vi "strain_fgv_config.vi"(8 "error in":errorcluster caption="에러 입력") -> (0 "error out":errorcluster caption="에러 출력", 3 "task out":refnum<k21> caption="태스크 출력")   [LabVIEW 2013]
uses:
  <vilib>/DAQmx/configure/timing.llb/DAQmx Timing (Sample Clock).vi
  <vilib>/DAQmx/create/channels.llb/DAQmx Create Channel (AI-Strain-Strain Gage).vi
  <resource>/objmgr/daqmx.rc
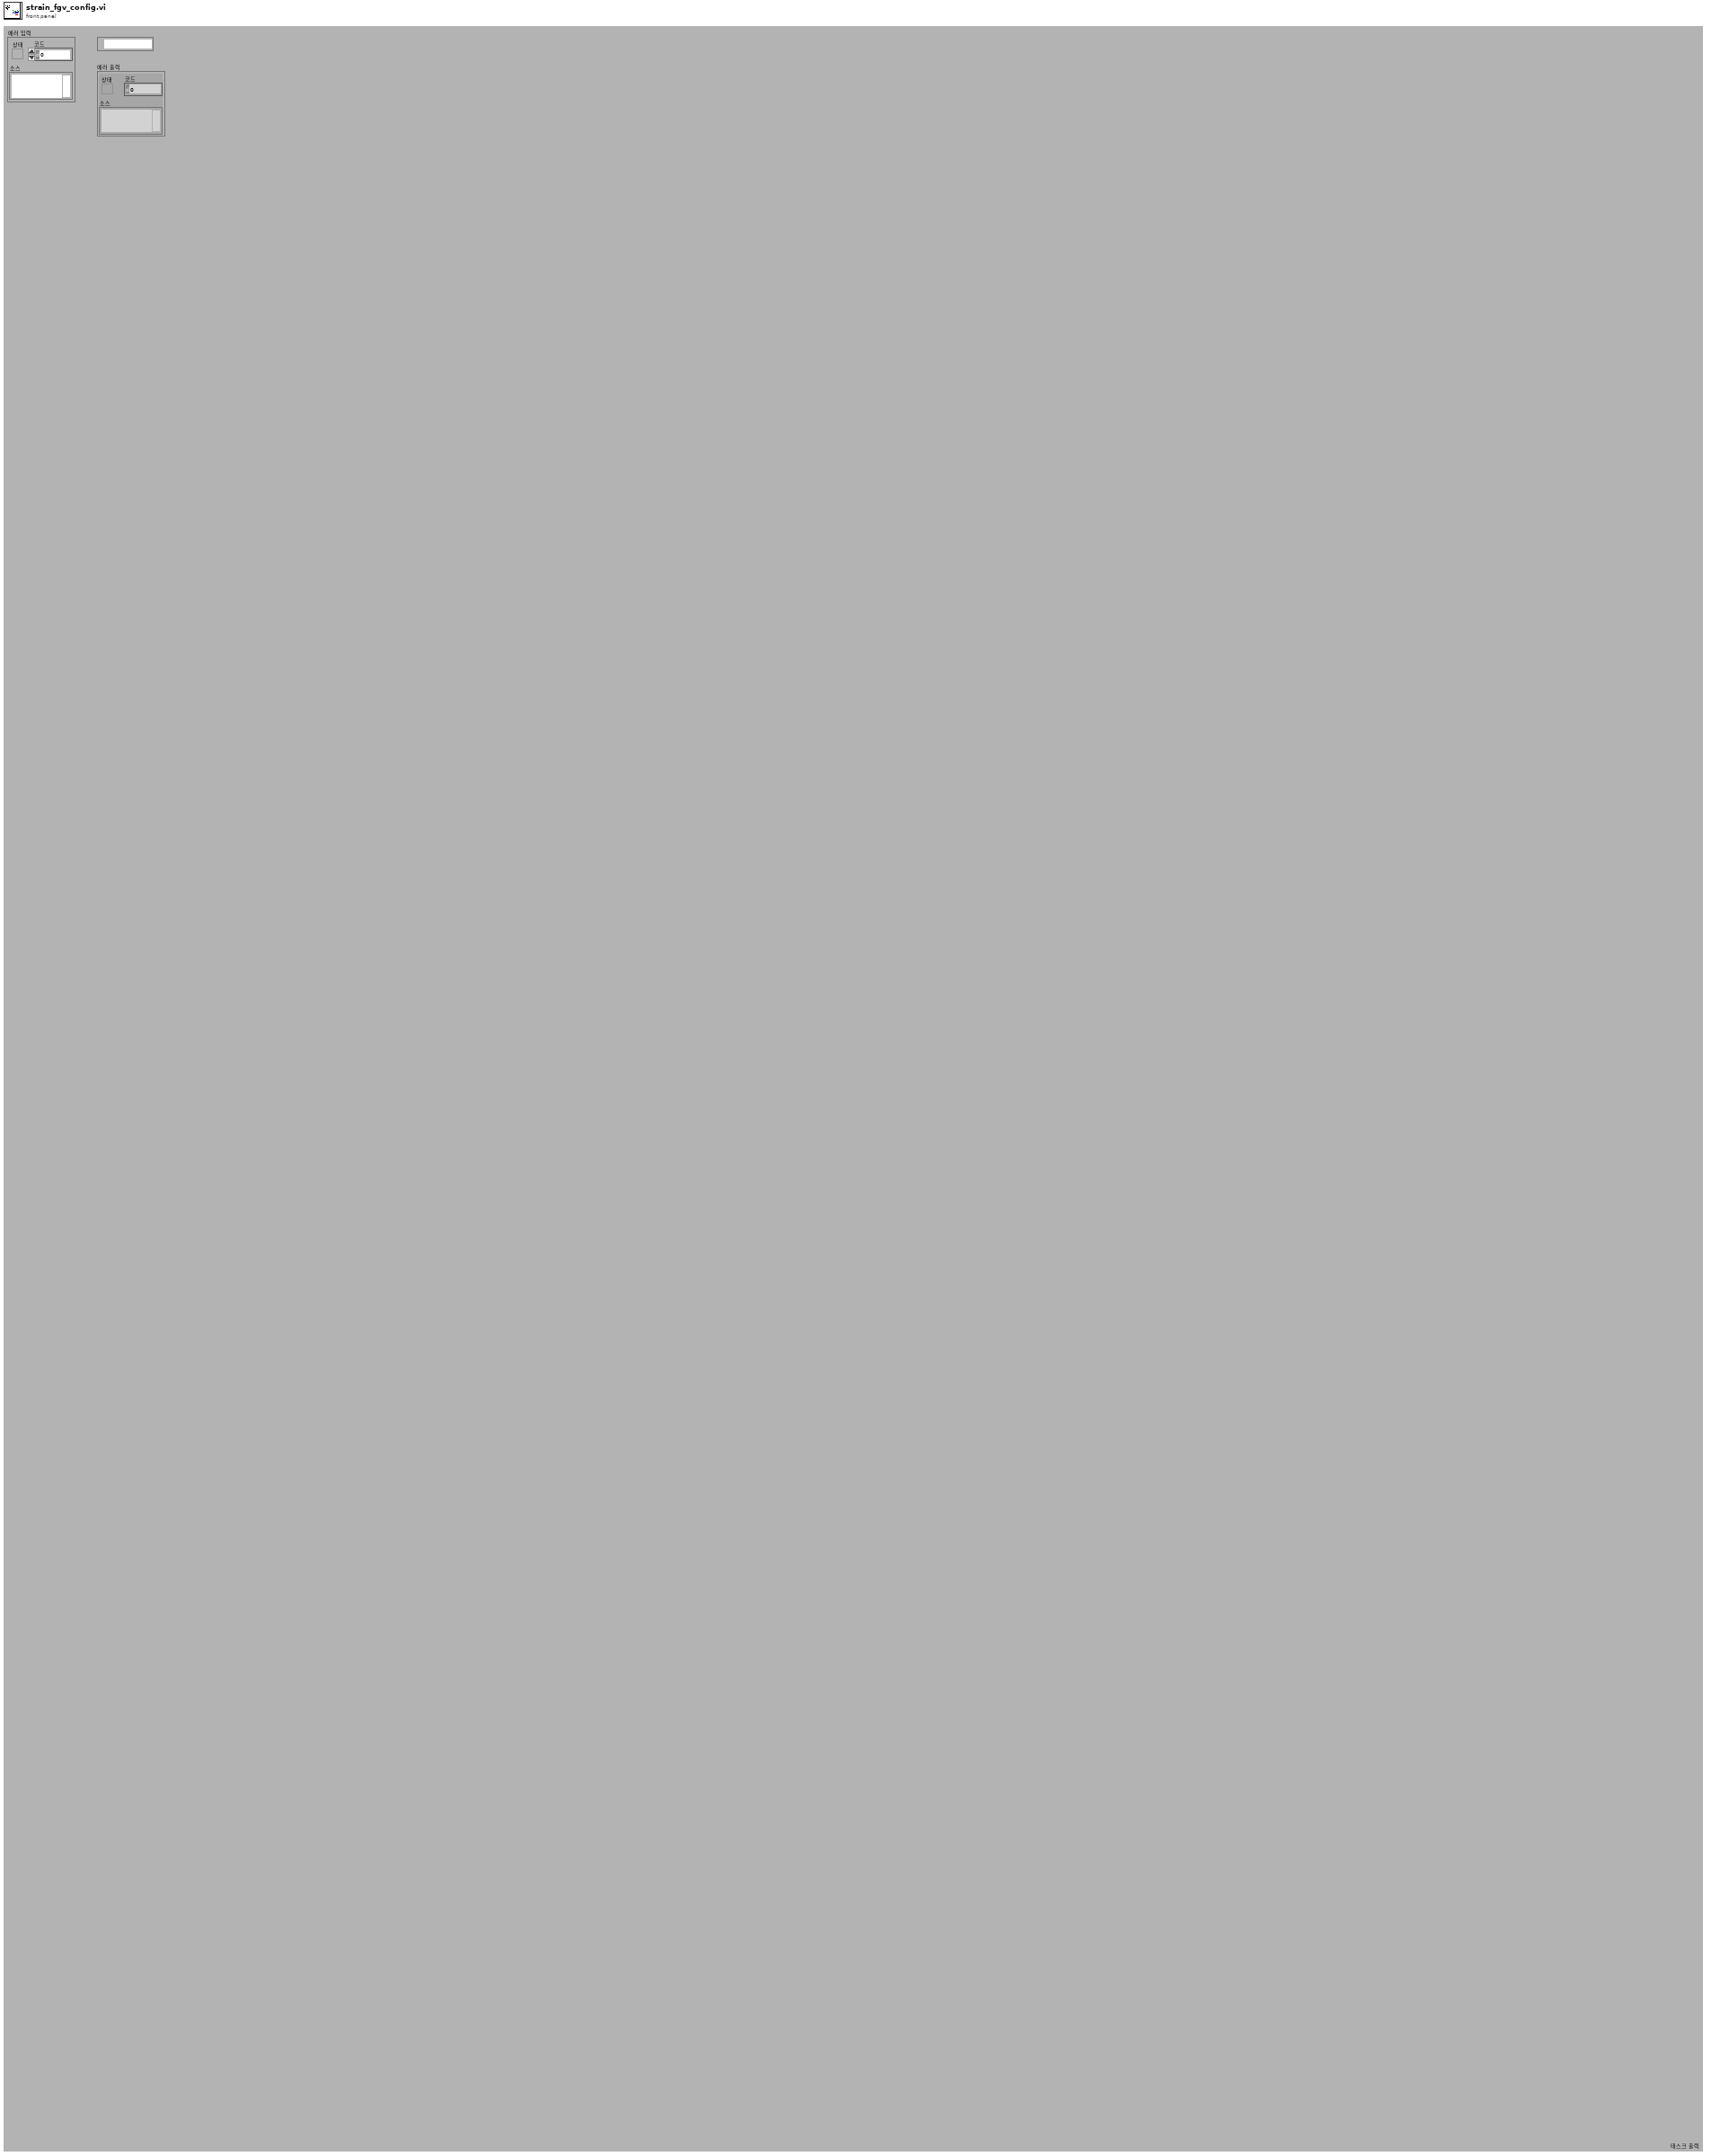
[diagram p1: front panel]
types:
  T1 = cluster{"strain configuration":i32, "lead resistance":dbl, "initial bridge voltage":dbl, "excitation source":i32, "excitation value":dbl}
  T2 = cluster{"gage factor":dbl, "nominal gage resistance":dbl, "poisson ratio":dbl}
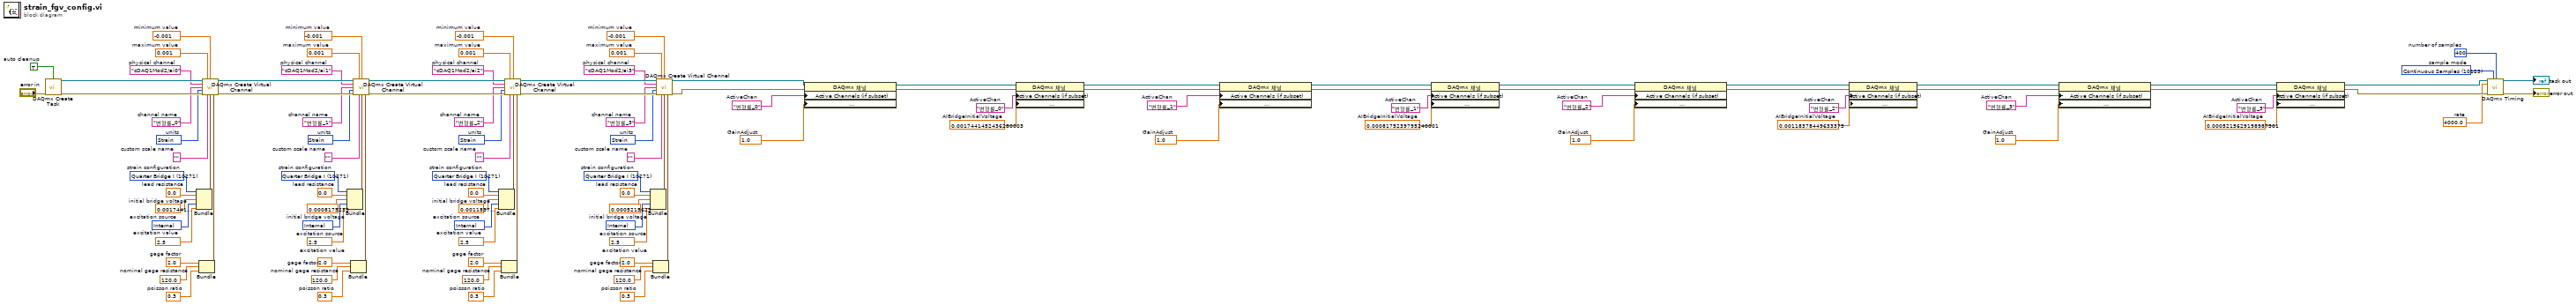
[diagram p0: block diagram]
diagram:
  w1 = 10123 items=["Finite Samples"=10178, "Continuous Samples"=10123, "Hardware Timed Single Point"=12522]  # sample mode
  w2 = 400  # number of samples
  w3 = 4000.0  # rate
  w7 = 0.0005215629198987501  # AIBridgeInitialVoltage
  w10 = "변형률_3"  # ActiveChan
  w11 = 1.0  # GainAdjust
  w14 = "변형률_3"  # ActiveChan
  w15 = 0.00118378449633375  # AIBridgeInitialVoltage
  w18 = "변형률_2"  # ActiveChan
  w19 = 1.0  # GainAdjust
  w22 = "변형률_2"  # ActiveChan
  w23 = 0.0008175239795240001  # AIBridgeInitialVoltage
  w26 = "변형률_1"  # ActiveChan
  w27 = 1.0  # GainAdjust
  w30 = "변형률_1"  # ActiveChan
  w31 = 0.0017441452436280003  # AIBridgeInitialVoltage
  w34 = "변형률_0"  # ActiveChan
  w35 = 1.0  # GainAdjust
  w38 = "변형률_0"  # ActiveChan
  w43 = 0.0  # lead resistance
  w46 = 0.3  # poisson ratio
  w42 = 0.0005215629198987501  # initial bridge voltage
  w47 = 120.0  # nominal gage resistance
  w45 = 2.0  # gage factor
  w40 = 2.5  # excitation value
  w41 = 10200 items=["Internal"=10200, "External"=10167, "None"=10230]  # excitation source
  w44 = 10271 items=["Full Bridge I"=10183, "Full Bridge II"=10184, "Full Bridge III"=10185, "Half Bridge I"=10188, "Half Bridge II"=10189, "Quarter Bridge I"=10271, "Quarter Bridge II"=10272]  # strain configuration
  w49 = 10299 items=["Strain"=10299, "From Custom Scale"=10065]  # units
  w50 = "변형률_3"  # channel name
  w52 = ""  # custom scale name
  w53 = -0.001  # minimum value
  w54 = 0.001  # maximum value
  w55 = "cDAQ1Mod2/ai3"  # physical channel
  w61 = 0.0  # lead resistance
  w64 = 0.3  # poisson ratio
  w60 = 0.00118378449633375  # initial bridge voltage
  w65 = 120.0  # nominal gage resistance
  w63 = 2.0  # gage factor
  w58 = 2.5  # excitation value
  w59 = 10200 items=["Internal"=10200, "External"=10167, "None"=10230]  # excitation source
  w62 = 10271 items=["Full Bridge I"=10183, "Full Bridge II"=10184, "Full Bridge III"=10185, "Half Bridge I"=10188, "Half Bridge II"=10189, "Quarter Bridge I"=10271, "Quarter Bridge II"=10272]  # strain configuration
  w67 = 10299 items=["Strain"=10299, "From Custom Scale"=10065]  # units
  w68 = "변형률_2"  # channel name
  w70 = ""  # custom scale name
  w71 = -0.001  # minimum value
  w72 = 0.001  # maximum value
  w73 = "cDAQ1Mod2/ai2"  # physical channel
  w79 = 0.0  # lead resistance
  w82 = 0.3  # poisson ratio
  w78 = 0.0008175239795240001  # initial bridge voltage
  w83 = 120.0  # nominal gage resistance
  w81 = 2.0  # gage factor
  w76 = 2.5  # excitation value
  w77 = 10200 items=["Internal"=10200, "External"=10167, "None"=10230]  # excitation source
  w80 = 10271 items=["Full Bridge I"=10183, "Full Bridge II"=10184, "Full Bridge III"=10185, "Half Bridge I"=10188, "Half Bridge II"=10189, "Quarter Bridge I"=10271, "Quarter Bridge II"=10272]  # strain configuration
  w85 = 10299 items=["Strain"=10299, "From Custom Scale"=10065]  # units
  w86 = "변형률_1"  # channel name
  w88 = ""  # custom scale name
  w89 = -0.001  # minimum value
  w90 = 0.001  # maximum value
  w91 = "cDAQ1Mod2/ai1"  # physical channel
  w97 = 0.0  # lead resistance
  w100 = 0.3  # poisson ratio
  w96 = 0.0017441452436280003  # initial bridge voltage
  w101 = 120.0  # nominal gage resistance
  w99 = 2.0  # gage factor
  w94 = 2.5  # excitation value
  w95 = 10200 items=["Internal"=10200, "External"=10167, "None"=10230]  # excitation source
  w98 = 10271 items=["Full Bridge I"=10183, "Full Bridge II"=10184, "Full Bridge III"=10185, "Half Bridge I"=10188, "Half Bridge II"=10189, "Quarter Bridge I"=10271, "Quarter Bridge II"=10272]  # strain configuration
  w103 = 10299 items=["Strain"=10299, "From Custom Scale"=10065]  # units
  w104 = "변형률_0"  # channel name
  w106 = ""  # custom scale name
  w107 = -0.001  # minimum value
  w108 = 0.001  # maximum value
  w109 = "cDAQ1Mod2/ai0"  # physical channel
  w111 = TRUE  # auto cleanup
  n1 = call <vilib>:"DAQmx Create Task.vi"("auto cleanup"=w111, "error in"="error in") -> ("task out"=w110:refnum<k21>, "error out"=w112:errorcluster)  [unwired: 12 in]
  n2 = Bundle("strain configuration"=w98, "lead resistance"=w97, "initial bridge voltage"=w96, "excitation source"=w95, "excitation value"=w94) -> (w93:T1)  [unwired: 1 in]
  n3 = Bundle("gage factor"=w99, "nominal gage resistance"=w101, "poisson ratio"=w100) -> (w102:T2)  [unwired: 1 in]
  n4 = call-poly <vilib>:"DAQmx Create Virtual Channel.vi"("task in"=w110, "maximum value"=w108, "minimum value"=w107, "physical channels"=w109, "name to assign"=w104, "units"=w103, "error in"=w112, "custom scale name"=w106, "bridge information"=w93, "strain gage information"=w102) -> ("task out"=w92:refnum<k21>, "error out"=w105:errorcluster)  [unwired: 4 in]
  n5 = Bundle("strain configuration"=w80, "lead resistance"=w79, "initial bridge voltage"=w78, "excitation source"=w77, "excitation value"=w76) -> (w75:T1)  [unwired: 1 in]
  n6 = Bundle("gage factor"=w81, "nominal gage resistance"=w83, "poisson ratio"=w82) -> (w84:T2)  [unwired: 1 in]
  n7 = call-poly <vilib>:"DAQmx Create Virtual Channel.vi"("task in"=w92, "maximum value"=w90, "minimum value"=w89, "physical channels"=w91, "name to assign"=w86, "units"=w85, "error in"=w105, "custom scale name"=w88, "bridge information"=w75, "strain gage information"=w84) -> ("task out"=w74:refnum<k21>, "error out"=w87:errorcluster)  [unwired: 4 in]
  n8 = Bundle("strain configuration"=w62, "lead resistance"=w61, "initial bridge voltage"=w60, "excitation source"=w59, "excitation value"=w58) -> (w57:T1)  [unwired: 1 in]
  n9 = Bundle("gage factor"=w63, "nominal gage resistance"=w65, "poisson ratio"=w64) -> (w66:T2)  [unwired: 1 in]
  n10 = call-poly <vilib>:"DAQmx Create Virtual Channel.vi"("task in"=w74, "maximum value"=w72, "minimum value"=w71, "physical channels"=w73, "name to assign"=w68, "units"=w67, "error in"=w87, "custom scale name"=w70, "bridge information"=w57, "strain gage information"=w66) -> ("task out"=w56:refnum<k21>, "error out"=w69:errorcluster)  [unwired: 4 in]
  n11 = Bundle("strain configuration"=w44, "lead resistance"=w43, "initial bridge voltage"=w42, "excitation source"=w41, "excitation value"=w40) -> (w39:T1)  [unwired: 1 in]
  n12 = Bundle("gage factor"=w45, "nominal gage resistance"=w47, "poisson ratio"=w46) -> (w48:T2)  [unwired: 1 in]
  n13 = call-poly <vilib>:"DAQmx Create Virtual Channel.vi"("task in"=w56, "maximum value"=w54, "minimum value"=w53, "physical channels"=w55, "name to assign"=w50, "units"=w49, "error in"=w69, "custom scale name"=w52, "bridge information"=w39, "strain gage information"=w48) -> ("task out"=w37:refnum<k21>, "error out"=w51:errorcluster)  [unwired: 4 in]
  n14 = property class="DAQmx 채널"(reference=w37, error in=w51, "Active Channels (if subset)"=w38, "Analog Input:General Properties:Signal Conditioning:Bridge:Shunt Cal:Gain Adjustment"=w35) -> (reference out=w32:refnum<k21>, error out=w36:errorcluster)
  n15 = property class="DAQmx 채널"(reference=w32, error in=w36, "Active Channels (if subset)"=w34, "Analog Input:General Properties:Signal Conditioning:Bridge:Initial Bridge Voltage"=w31) -> (reference out=w29:refnum<k21>, error out=w33:errorcluster)
  n16 = property class="DAQmx 채널"(reference=w29, error in=w33, "Active Channels (if subset)"=w30, "Analog Input:General Properties:Signal Conditioning:Bridge:Shunt Cal:Gain Adjustment"=w27) -> (reference out=w24:refnum<k21>, error out=w28:errorcluster)
  n17 = property class="DAQmx 채널"(reference=w24, error in=w28, "Active Channels (if subset)"=w26, "Analog Input:General Properties:Signal Conditioning:Bridge:Initial Bridge Voltage"=w23) -> (reference out=w21:refnum<k21>, error out=w25:errorcluster)
  n18 = property class="DAQmx 채널"(reference=w21, error in=w25, "Active Channels (if subset)"=w22, "Analog Input:General Properties:Signal Conditioning:Bridge:Shunt Cal:Gain Adjustment"=w19) -> (reference out=w16:refnum<k21>, error out=w20:errorcluster)
  n19 = property class="DAQmx 채널"(reference=w16, error in=w20, "Active Channels (if subset)"=w18, "Analog Input:General Properties:Signal Conditioning:Bridge:Initial Bridge Voltage"=w15) -> (reference out=w13:refnum<k21>, error out=w17:errorcluster)
  n20 = property class="DAQmx 채널"(reference=w13, error in=w17, "Active Channels (if subset)"=w14, "Analog Input:General Properties:Signal Conditioning:Bridge:Shunt Cal:Gain Adjustment"=w11) -> (reference out=w8:refnum<k21>, error out=w12:errorcluster)
  n21 = property class="DAQmx 채널"(reference=w8, error in=w12, "Active Channels (if subset)"=w10, "Analog Input:General Properties:Signal Conditioning:Bridge:Initial Bridge Voltage"=w7) -> (reference out=w4:refnum<k21>, error out=w9:errorcluster)
  n22 = call-poly <vilib>:"DAQmx Timing.vi"("task/channels in"=w4, "sample mode"=w1, "samples per channel"=w2, "rate"=w3, "error in"=w9) -> ("task out"=→"task out":refnum<k21>, "error out"=→"error out":errorcluster)  [unwired: 9 in]
